vi "N9030B_0912.vi"() -> ()   [LabVIEW 2017]
uses:
  <vilib>/Utility/file.llb/Write Delimited Spreadsheet (DBL).vi
  <instrlib>/Keysight XSAn/Keysight XSAn.lvlib
panel:
  out "element":dbl
  out "sweep":bool
  in  "stop":bool
  in  "Path":path=path "d:/"
  out "frequency 3":cluster{"X":dbl, "Y":dbl}[](graph)
  out "actual points":i32
  in  "Array":cluster{"Numeric":dbl, "Numeric 2":dbl}[](array[cluster])
  out "frequency 2":cluster{"X":dbl, "Y":dbl}[](graph)
  in  "frequency points (1 is reference)":T1 {"frequency 3 (Hz)" format="%#_6p"; "frequency 2 (Hz)" format="%#_6p"; "frequency 1 (Hz)" format="%#_6p"}
  in  "Keysight N9030B":refnum<visa-resource-name> caption="resource name"
  in  "Rigol DG5252":refnum<visa-resource-name>
  in  "Rigol DG5252":T2={"start frequency (MHz)"=150.0, "frequency spacing (MHz)"=1.0, "stop frequency (MHz)"=250.0, "sweep frequency"=FALSE}
  out "error out":errorcluster {"code" format="%.0x"}
  in  "Keysight N9030B":T3={"resolution bandwidth"=3.0, "video bandwidth"=3.0, "center frequency"=15000.0, "span"=5000.0, "option string"=""} {"span" format="%#_6p"; "center frequency" format="%#_6p"; "video bandwidth" format="%#_6p"; "resolution bandwidth" format="%#_6p"}
  out "amplitude":dbl[](array[numeric])
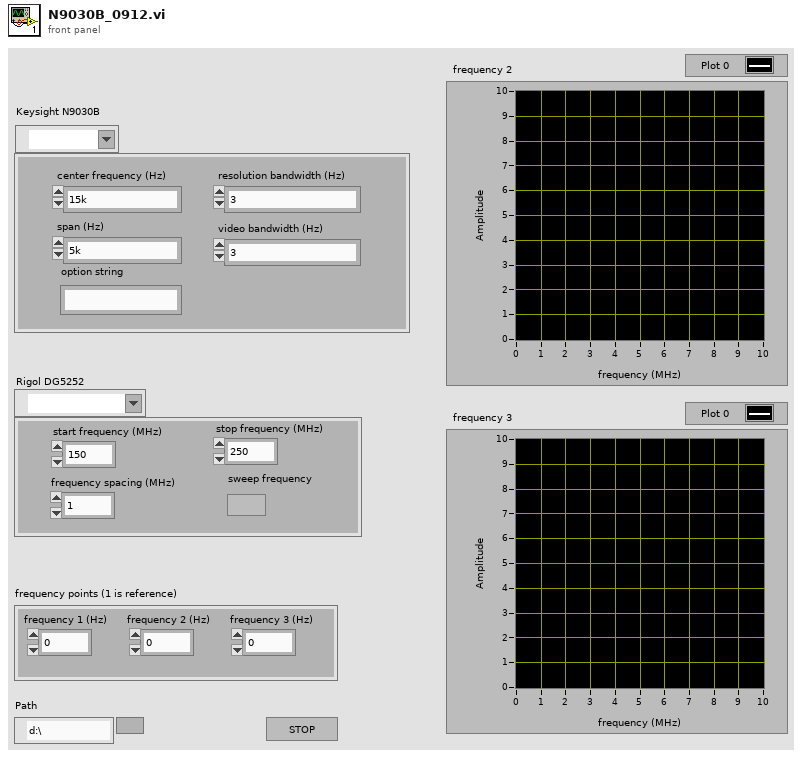
[diagram p1: front panel]
types:
  T1 = cluster{"frequency 1 (Hz)":dbl, "frequency 2 (Hz)":dbl, "frequency 3 (Hz)":dbl}
  T2 = cluster{"start frequency (MHz)":dbl, "frequency spacing (MHz)":dbl, "stop frequency (MHz)":dbl, "sweep frequency":bool}
  T3 = cluster{"resolution bandwidth":dbl, "video bandwidth":dbl, "center frequency":dbl, "span":dbl, "option string":string}
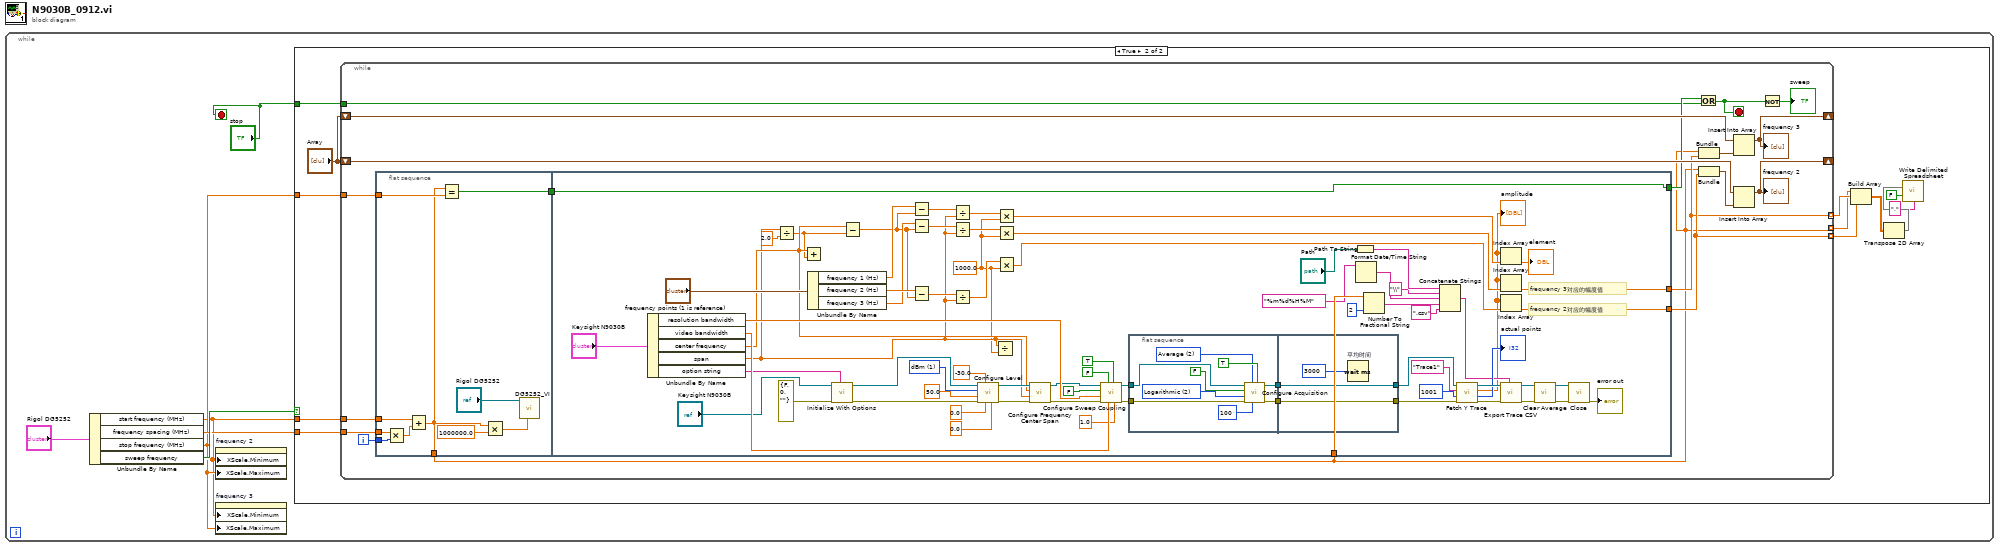
[diagram p0: block diagram]
diagram:
  n1 = while {
    stop <- "stop" stop-if-true
    n2 = Unbundle By Name("Rigol DG5252") -> ("start frequency (MHz)"=w2:dbl, "frequency spacing (MHz)"=w4:dbl, "stop frequency (MHz)"=w3:dbl, "sweep frequency"=w5:bool)
    n3 = property on="frequency 2" class="XYGraph (strict)"("XScale.Minimum"=w2, "XScale.Maximum"=w3) -> ()  [unwired: 2 in, 2 out]
    n4 = property on="frequency 3" class="XYGraph (strict)"("XScale.Minimum"=w2, "XScale.Maximum"=w3) -> ()  [unwired: 2 in, 2 out]
    n5 = case shown="True" w5 {
      tunnel: w2 -> [_ w16]
      tunnel: w4 -> [_ w18]
      tunnel: w3 -> [_ w15]
      tunnel: "stop" -> [_ w10]
      frame False {
      }
      frame True {
        n6 = while {
          tunnel: w16 -> [w36]
          tunnel: w18 -> [w35]
          tunnel: w15 -> [w33]
          shift-right: [w26] -> _
          shift-left: "Array" -> [w31]
          shift-right: [w28] -> _
          shift-left: "Array" -> [w30]
          tunnel: [w22] -> w11 mode=indexing
          tunnel: [w21] -> w14 mode=indexing
          tunnel: [w20] -> w13 mode=indexing
          tunnel: w10 -> [w19]
          i -> [w34]
          stop <- w24 stop-if-true
          n7 = flat-sequence {
            tunnel: w36 -> [w45]
            tunnel: w35 -> [w44]
            tunnel: w34 -> [w43]
            tunnel: w33 -> [w39]
            tunnel: [w38] -> w32
            tunnel: [w37] -> w20
            tunnel: [w117] -> w25
            tunnel: w32 -> [w117]
            tunnel: [w103] -> w22
            tunnel: [w102] -> w21
            tunnel: w20 -> [w61]
            frame #0 {
              n8 = Multiply(x=w44, y=w43) -> (x*y=w42:dbl)
              n9 = Add(x=w45, y=w42) -> (x+y=w37:dbl)
              n10 = Equal?(x=w37, y=w39) -> (x = y?=w38:bool)
              n11 = Multiply(x=w37, y=1000000.0) -> (x*y=w40:dbl)
              n12 = call "DG5252_VI.vi"("Frequency (1000 Hz)"=w40, "VISA resource name"="Rigol DG5252") -> ()  [unwired: 10 in]
            }
            frame #1 {
              w50 = 1000.0 ("y")
              w94 = 1 items=["dBm"=1, "dBmV"=2, "dBuV"=3, "Volt"=4, "Watt"=5] ("amplitude units (dBm)")
              # "frequency 3对应的幅度值"
              # "frequency 2对应的幅度值"
              n13 = Unbundle By Name("Keysight N9030B") -> ("resolution bandwidth"=w113:dbl, "video bandwidth"=w115:dbl, "center frequency"=w75:dbl, "span"=w52:dbl, "option string"=w114:string)
              n14 = Divide(x=w52, y=2.0) -> (x/y=w74:dbl)
              n15 = Add(x=w75, y=w74) -> ()  [unwired: 1 out]
              n16 = Unbundle By Name("frequency points (1 is reference)") -> ("frequency 1 (Hz)"=w55:dbl, "frequency 2 (Hz)"=w73:dbl, "frequency 3 (Hz)"=w69:dbl)
              n17 = call <instrlib>:"Initialize With Options.vi"("option string"=w114, "error in (no error)"=errorcluster {"status"=FALSE, "code"=0, "source"=""}, "resource string"="Keysight N9030B") -> ("error out"=w97:errorcluster, "instrument handle out"=w98:refnum<k15>)  [unwired: 7 in]
              n18 = Subtract(x=w75, y=w74) -> (x-y=w54:dbl)
              n19 = Subtract(x=w55, y=w54) -> (x-y=w53:dbl)
              n20 = Subtract(x=w69, y=w54) -> (x-y=w68:dbl)
              n21 = Subtract(x=w73, y=w54) -> (x-y=w72:dbl)
              n22 = Divide(x=w53, y=w52) -> (x/y=w51:dbl)
              n23 = Divide(x=w68, y=w52) -> (x/y=w67:dbl)
              n24 = Divide(x=w72, y=w52) -> (x/y=w71:dbl)
              n25 = call <instrlib>:"Configure Level.vi"("attenuation"=0.0, "reference level offset"=0.0, "reference level"=-30.0, "error in (no error)"=w97, "input impedance"=50.0, "amplitude units (dBm)"=w94, "instrument handle"=w98) -> ("error out"=w101:errorcluster, "instrument handle out"=w100:refnum<k15>)  [unwired: 3 in]
              n26 = Divide(x=w52, y=w50) -> ()  [unwired: 1 out]
              n27 = Multiply(x=w51, y=w50) -> (x*y=w49:dbl)
              n28 = Multiply(x=w67, y=w50) -> (x*y=w66:dbl)
              n29 = Multiply(x=w71, y=w50) -> (x*y=w70:dbl)
              n30 = call <instrlib>:"Configure Frequency Center Span.vi"("error in (no error)"=w101, "span"=w52, "center frequency"=w75, "instrument handle"=w100) -> ("error out"=w109:errorcluster, "instrument handle out"=w108:refnum<k15>)  [unwired: 6 in]
              n31 = call <instrlib>:"Configure Sweep Coupling.vi"("sweep time"=1.0, "sweep time auto (Off)"=TRUE, "video bandwidth"=w115, "video bandwidth auto (Off)"=FALSE, "error in (no error)"=w109, "resolution bandwidth"=w113, "resolution bandwidth auto (Off)"=FALSE, "instrument handle"=w108) -> ("error out"=w87:errorcluster, "instrument handle out"=w86:refnum<k15>)  [unwired: 2 in]
              n32 = flat-sequence {
                tunnel: w87 -> [w123]
                tunnel: w86 -> [w126]
                tunnel: [w125] -> w78
                tunnel: [w124] -> w77
                tunnel: [w128] -> w84
                tunnel: [w129] -> w85
                tunnel: w78 -> [w129]
                tunnel: w77 -> [w128]
                frame #0 {
                  w120 = 2 items=["Auto Peak"=1, "Average"=2, "Maximum Peak"=3, "Minimum Peak"=4, "Sample"=5, "RMS"=6] ("detector type (Auto Peak)")
                  w122 = 2 items=["Linear"=1, "Logarithmic"=2] ("vertical scale (Linear)")
                  n33 = call <instrlib>:"Configure Acquisition.vi"("sweep mode continuous (Off)"=TRUE, "number of sweeps"=100, "detector type (Auto Peak)"=w120, "error in (no error)"=w123, "vertical scale (Linear)"=w122, "detector type auto (Off)"=FALSE, "instrument handle"=w126) -> ("error out"=w124:errorcluster, "instrument handle out"=w125:refnum<k15>)  [unwired: 3 in]
                }
                frame #1 {
                  n34 = Wait (ms) "平均时间"(milliseconds to wait=u32 3000) -> ()  [unwired: 1 out]
                }
              }
              n35 = Path To String(path="Path") -> (string=w64:string)
              n36 = Format Date/Time String(time format string (%c)="%m%d%H%M") -> (date/time string=w56:string)  [unwired: 2 in]
              n37 = Number To Fractional String(number=w61, precision (6)=i16 2) -> (F-format string=w60:string)  [unwired: 2 in]
              n38 = Concatenate Strings(w64, "\\" ("string"), w56, w60, ".csv" ("string")) -> (w58:string)
              n39 = call <instrlib>:"Fetch Y Trace.vi"("error in (no error)"=w84, "array length"=1001, "trace name"="Trace1", "instrument handle"=w85) -> ("error out"=w111:errorcluster, "actual points"=→"actual points":i32, "amplitude"=w48:dbl[], "instrument handle out"=w110:refnum<k15>)  [unwired: 4 in]
              "amplitude" <- w48
              n40 = Index Array(array=w48, index=w49) -> (element=→"element":dbl)
              n41 = Index Array(array=w48, index=w66) -> (element=w102:dbl)
              n42 = Index Array(array=w48, index=w70) -> (element=w103:dbl)
              n43 = call <instrlib>:"Export Trace CSV.vi"("Filename"=w58, "error in (no error)"=w111, "instrument handle"=w110) -> ("error out"=w81:errorcluster, "instrument handle out"=w82:refnum<k15>)  [unwired: 7 in]
              n44 = call <instrlib>:"Clear Average.vi"("error in (no error)"=w81, "instrument handle"=w82) -> ("error out"=w79:errorcluster, "instrument handle out"=w80:refnum<k15>)  [unwired: 8 in]
              n45 = call <instrlib>:"Close.vi"("error in (no error)"=w79, "instrument handle"=w80) -> ("error out"=→"error out":errorcluster)  [unwired: 9 in]
            }
          }
          n46 = Or(x=w25, y=w19) -> (x .or. y?=w24:bool)
          n47 = Bundle(w20, "amplitude 2"=w21) -> (w27:cluster{dbl, "amplitude 2":dbl})  [unwired: 1 in]
          n48 = Bundle(w20, "amplitude 2"=w22) -> (w29:cluster{dbl, "amplitude 2":dbl})  [unwired: 1 in]
          n49 = Insert Into Array(array=w31, new element=w27) -> (w26:cluster{"Numeric":dbl, "Numeric 2":dbl}[])  [unwired: 1 in]
          "frequency 3" <- w26
          n50 = Insert Into Array(array=w30, new element=w29) -> (w28:cluster{"Numeric":dbl, "Numeric 2":dbl}[])  [unwired: 1 in]
          "frequency 2" <- w28
          n51 = Not(x=w24) -> (.not. x?=→"sweep":bool)
        }
        n52 = Build Array(w13, w14, w11) -> (w9:dbl[][])
        n53 = Transpose 2D Array(2D array=w9) -> (transposed array=w8:dbl[][])
        n54 = call-poly <vilib>:"Write Delimited Spreadsheet.vi"("2D data"=w8, "append to file? (new file:F)"=FALSE, "delimiter (\\t)"="," ("delimiter (\\t)")) -> ()  [unwired: 11 in, 2 out]
      }
    }
  }
